vi "_emi_SMLoop Control Array.vi"(5 "Loop IDs":u16[](array[numeric]), 7 "Enable":bool, 9 "error in (no error)":errorcluster) -> (6 "Loop IDs out":u16[](array[numeric]), 10 "error out":errorcluster)   [LabVIEW 2011]
doc: "Set the wanted execution state of a SMLoop."
uses:
  Loop control/Private/_emi_GFV Loop Linking.vi
  Loop control/Private/_emi_GFV Loop Enable.vi
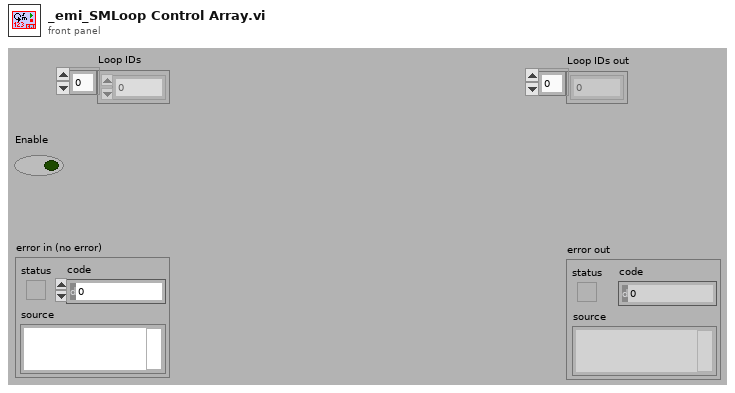
[diagram p1: front panel]
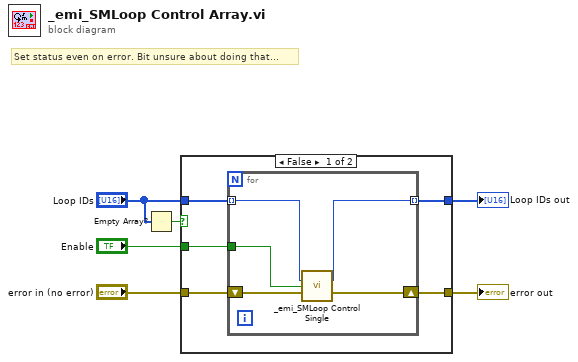
[diagram p0: block diagram]
diagram:
  # "Set status even on error. Bit unsure about doing that..."
  n1 = Empty Array?(array="Loop IDs") -> (empty?=w6:bool)
  n2 = case shown="False" w6 {
    tunnel: "Loop IDs" -> [w9 w17]
    tunnel: "error in (no error)" -> [w11 w18]
    tunnel: [w10 w18] -> w4
    tunnel: [w8 w17] -> w1
    tunnel: "Enable" -> [w7 _]
    frame False {
      n3 = for {
        shift-right: [w15] -> w10
        shift-left: w11 -> [w16]
        tunnel: w9 -> [w14] mode=indexing
        tunnel: [w13] -> w8 mode=indexing
        tunnel: w7 -> [w12]
        n4 = call "_emi_SMLoop Control Single.vi"("Loop ID in"=w14, "Enable"=w12, "error in (no error)"=w16) -> ("Loop ID out"=w13:u16, "error out"=w15:errorcluster)  [unwired: 11 in]
      }
    }
    frame True {
    }
  }
  "error out" <- w4
  "Loop IDs out" <- w1
